vi "Destroy Timer IRQ.vi"(8 "error in (no error)":errorcluster, 11 "Timer ID":u8) -> (0 "error out":errorcluster)   [LabVIEW 2021, in "Timer IRQ.lvlib"]
doc: "Destroys timer interrupts. After you destroy an interrupt, LabVIEW stops creating the interrupt and releases the resources associated with the interrupt."
uses:
  <vilib>/myRIO/Instrument Drivers/IRQ/Timer IRQ/Timer IRQ.lvlib
  <vilib>/myRIO/Common/Instrument Driver Framework/Utilities/typedefs/FPGA Ref Manager Action Enum.ctl
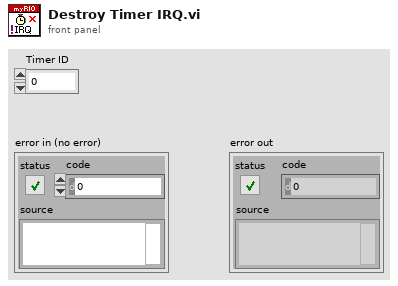
[diagram p1: front panel]
types:
  T1 = typedef "FPGA Ref Manager Action Enum.ctl" = enum16{"Get", "Set", "Reset"}
  T2 = typedef "Generic FPGA Reference.ctl" = refnum<k20>
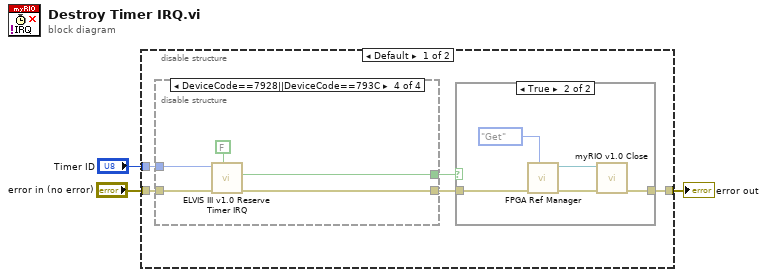
[diagram p0: block diagram]
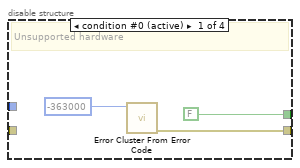
[diagram p2: hidden frame]
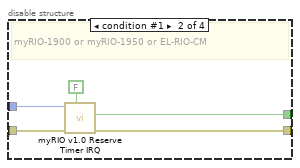
[diagram p3: hidden frame]
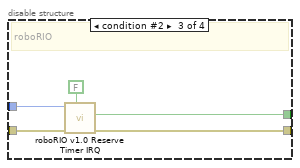
[diagram p4: hidden frame]
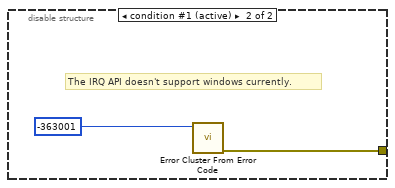
[diagram p6: hidden frame]
diagram:
  n1 = disable-structure shown="Default" {
    disable-tunnel: [w8 w33] -> w3
    disable-tunnel: "Timer ID" -> [w7 _]
    disable-tunnel: "error in (no error)" -> [w4 _]
    frame condition #0 {
      n2 = disable-structure shown="DeviceCode==7928||DeviceCode==793C" {
        disable-tunnel: w7 -> [_ w16 w21 w25]
        disable-tunnel: [w10 w15 w20 w22] -> w6
        disable-tunnel: [FALSE ("Succeed?") w14 w19 w23] -> w5
        disable-tunnel: w4 -> [_ w13 w18 w24]
        frame condition #0 (active) {
          # "Unsupported hardware"
          n3 = call <vilib>:"Error Cluster From Error Code.vi"("error code (0)"=-363000) -> ("error out"=w10:errorcluster)  [unwired: 8 in]
        }
        frame condition #1 {
          # "myRIO-1900 or myRIO-1950 or EL-RIO-CM"
          n4 = call <vilib>:"myRIO v1.0 Reserve Timer IRQ.vi"("Reserve?"=FALSE, "error in (no error)"=w13, "Timer ID"=w16) -> ("error out"=w15:errorcluster, "Succeed?"=w14:bool)  [unwired: 7 in]
        }
        frame condition #2 {
          # "roboRIO"
          n5 = call <vilib>:"roboRIO v1.0 Reserve Timer IRQ.vi"("Reserve?"=FALSE, "error in (no error)"=w18, "Timer ID"=w21) -> ("error out"=w20:errorcluster, "Succeed?"=w19:bool)  [unwired: 7 in]
        }
        frame condition #3 {
          n6 = call <vilib>:"ELVIS III v1.0 Reserve Timer IRQ.vi"("Reserve?"=FALSE, "error in (no error)"=w24, "Timer ID"=w25) -> ("error out"=w22:errorcluster, "Succeed?"=w23:bool)  [unwired: 7 in]
        }
      }
      n7 = case shown="True" w5 {
        tunnel: w6 -> [w27 w29]
        tunnel: [w27 w28] -> w8
        frame False {
        }
        frame True {
          n8 = call <vilib>:"FPGA Ref Manager.vi"("Action"=FPGA_Ref_Manager_Action_Enum."Get", "error in (no error)"=w29) -> ("error out"=w32:errorcluster, "Generic FPGA Reference out"=w31:T2)  [unwired: 7 in]
          n9 = call <vilib>:"myRIO v1.0 Close.vi"("error in (no error)"=w32, "myRIO FPGA Ref In"=w31) -> ("error out"=w28:errorcluster)  [unwired: 9 in]
        }
      }
    }
    frame condition #1 (active) {
      # "The IRQ API doesn't support windows currently."
      n10 = call <vilib>:"Error Cluster From Error Code.vi"("error code (0)"=-363001) -> ("error out"=w33:errorcluster)  [unwired: 8 in]
    }
  }
  "error out" <- w3
